vi "ReadEncoder.vi"() -> ()   [LabVIEW 2013]
doc: "This example demonstrates how to use a counter input along with an external clock to continually sample the angular position measured from an encoder.\n\nFor instructions on how to connect your signals to the DAQ device, refer to your device documentation."
uses:
  <vilib>/Utility/error.llb/DialogType.ctl
  <vilib>/DAQmx/read.llb/DAQmx Read (Counter 1D DBL 1Chan NSamp).vi
  <vilib>/DAQmx/create/channels.llb/DAQmx Create Channel (CI-Position-Angular Encoder).vi
  <vilib>/DAQmx/configure/timing.llb/DAQmx Timing (Sample Clock).vi
  <vilib>/DAQmx/create/channels.llb/DAQmx Create Channel (CO-Pulse Generation-Frequency).vi
  <vilib>/DAQmx/configure/timing.llb/DAQmx Timing (Implicit).vi
  <vilib>/DAQmx/miscellaneous.llb/DAQmx Fill In Error Info.vi
  <resource>/objmgr/daqmx.rc
panel:
  out "stop":bool=TRUE
  out "Waveform":waveform(dbl)(graph)={"t0"=timestamp(0 s since 1904-01-01), "dt"=0.001, "Y"=array[16000 elements]}
  out "CO.ActualDutyCycle":dbl=0.5
  out "CO.ActualFreq":dbl=10000.0
  in  "Output Terminal":tag="/Dev1/PFI12"
  in  "CounterOutput":tag="Dev1/ctr1"
  in  "Pulses Per Revolution":u32=200
  in  "EncodeCounterInput":tag="Dev1/ctr0"
  in  "Stop":bool
  in  "Sample Rate":dbl=1000.0
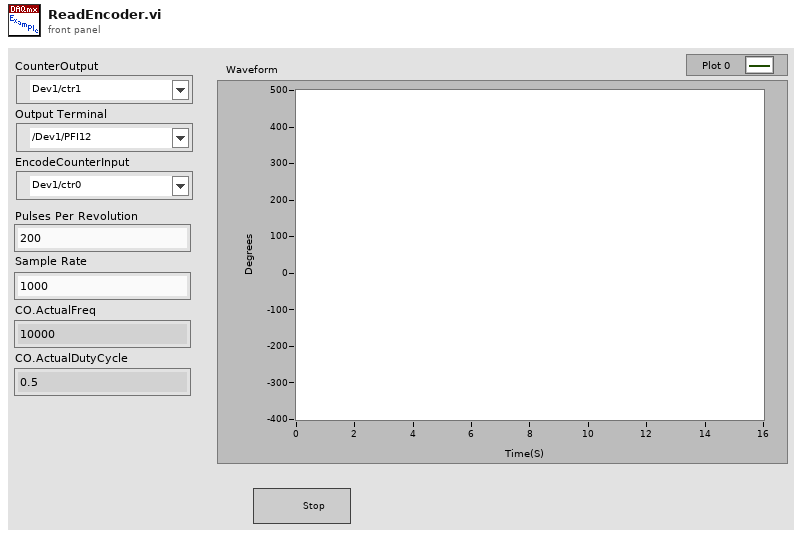
[diagram p1: front panel]
types:
  T1 = typedef "DialogType.ctl" = u16
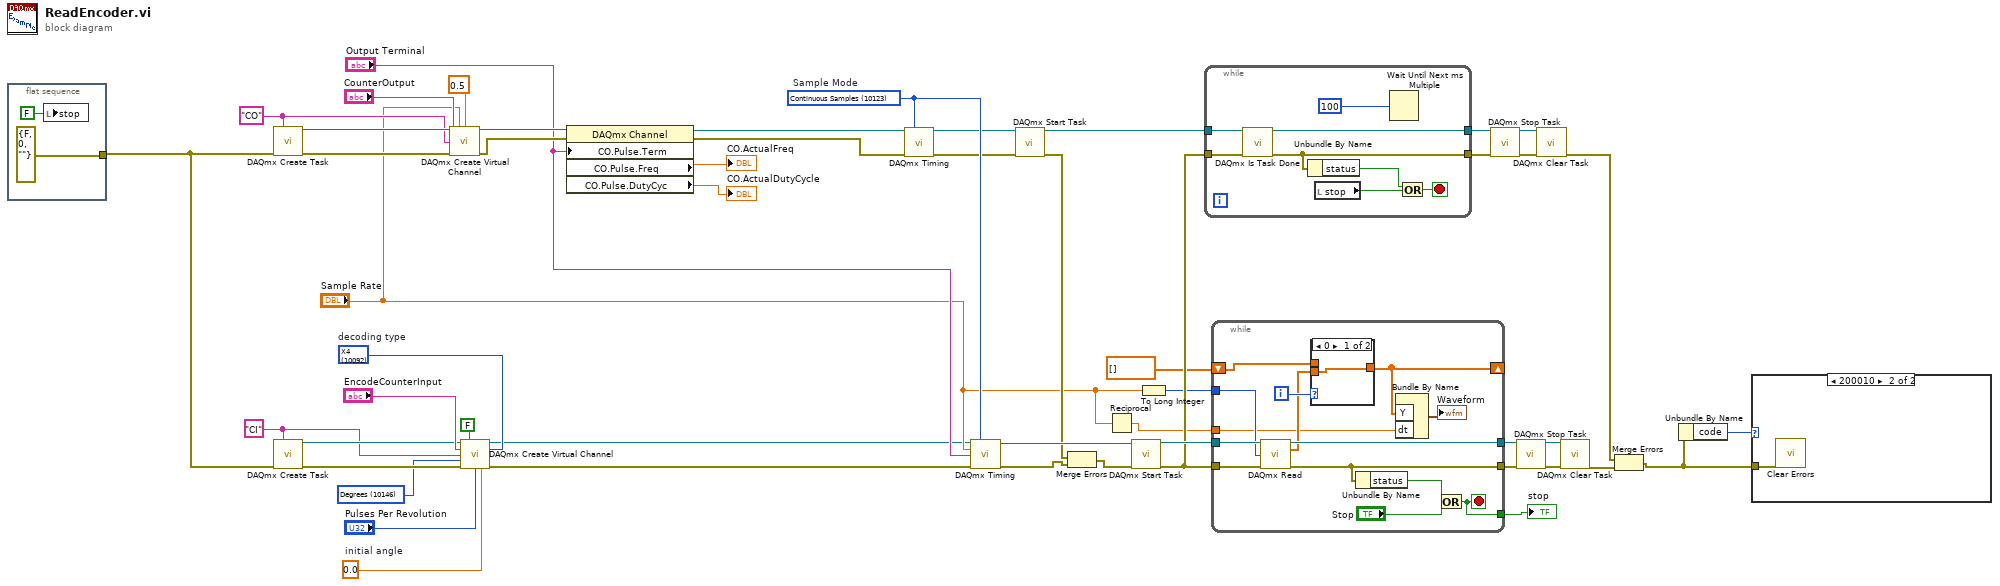
[diagram p0: block diagram]
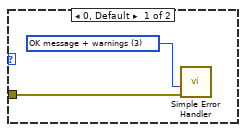
[diagram p2: hidden frame]
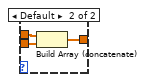
[diagram p3: hidden frame]
diagram:
  w4 = 0.0  # initial angle
  w5 = 10092 items=["X1"=10090, "X2"=10091, "X4"=10092, "Two Pulse Counting"=10313]  # decoding type
  w14 = 10146 items=["Degrees"=10146, "Radians"=10273, "Ticks"=10304, "From Custom Scale"=10065] ("units")
  w15 = "CI" ("new task name")
  w18 = "CO" ("new task name")
  w30 = 10123 items=["Finite Samples"=10178, "Continuous Samples"=10123, "Hardware Timed Single Point"=12522]  # Sample Mode
  n1 = flat-sequence {
    tunnel: [errorcluster {"status"=FALSE, "code"=0, "source"=""} ("error in")] -> w13
    frame #0 {
      n2 = local write "stop"(FALSE ("stop")) -> ()
    }
  }
  n3 = call <vilib>:"DAQmx Create Task.vi"("new task name"=w18, "error in"=w13) -> ("task out"=w20:refnum<k21>, "error out"=w19:errorcluster)  [unwired: 12 in]
  n4 = call <vilib>:"DAQmx Create Task.vi"("new task name"=w15, "error in"=w13) -> ("task out"=w16:refnum<k21>, "error out"=w17:errorcluster)  [unwired: 12 in]
  n5 = call-poly <vilib>:"DAQmx Create Virtual Channel.vi"("task in"=w20, "frequency"="Sample Rate", "duty cycle"=0.5 ("Duty Cycle"), "counter"="CounterOutput", "name to assign"=w18, "error in"=w19) -> ("task out"=w41:refnum<k21>, "error out"=w40:errorcluster)  [unwired: 8 in]
  n6 = call-poly <vilib>:"DAQmx Create Virtual Channel.vi"("task in"=w16, "z index enable"=FALSE ("Z Index Enable"), "counter"="EncodeCounterInput", "decoding type"=w5, "name to assign"=w15, "units"=w14, "error in"=w17, "pulses per revolution"="Pulses Per Revolution", "initial angle"=w4) -> ("task out"=w2:refnum<k21>, "error out"=w1:errorcluster)  [unwired: 5 in]
  n7 = property class="DAQmx Channel"(reference=w41, error in=w40, "CO.Pulse.Term"="Output Terminal") -> (reference out=w38:refnum<k21>, error out=w39:errorcluster, "CO.Pulse.Freq"=→"CO.ActualFreq":dbl, "CO.Pulse.DutyCyc"=→"CO.ActualDutyCycle":dbl)
  n8 = call-poly <vilib>:"DAQmx Timing.vi"("task/channels in"=w38, "sample mode"=w30, "error in"=w39) -> ("task out"=w29:refnum<k21>, "error out"=w28:errorcluster)  [unwired: 11 in]
  n9 = call-poly <vilib>:"DAQmx Timing.vi"("task/channels in"=w2, "sample mode"=w30, "rate"="Sample Rate", "source"="Output Terminal", "error in"=w1) -> ("task out"=w27:refnum<k21>, "error out"=w26:errorcluster)  [unwired: 9 in]
  n10 = call <vilib>:"DAQmx Start Task.vi"("task/channels in"=w29, "error in"=w28) -> ("task out"=w43:refnum<k21>, "error out"=w25:errorcluster)  [unwired: 12 in]
  n11 = Merge Errors(w25, w26) -> (w24:errorcluster)
  n12 = Reciprocal(x="Sample Rate") -> (1/x=w7:dbl)
  n13 = call <vilib>:"DAQmx Start Task.vi"("task/channels in"=w27, "error in"=w24) -> ("task out"=w51:refnum<k21>, "error out"=w23:errorcluster)  [unwired: 12 in]
  n14 = To Long Integer(number="Sample Rate") -> (32bit integer=w22:i32)
  n15 = while {
    tunnel: w43 -> [w61]
    tunnel: w23 -> [w60]
    tunnel: [w57] -> w31
    tunnel: [w58] -> w32
    stop <- w59 stop-if-true
    n16 = call <vilib>:"DAQmx Is Task Done.vi"("task/channels in"=w61, "error in"=w60) -> ("task out"=w58:refnum<k21>, "error out"=w57:errorcluster)  [unwired: 11 in, 1 out]
    n17 = Unbundle By Name(w57) -> ("status"=w56:bool)
    n18 = local read "stop"() -> (w54:bool)
    n19 = Wait Until Next ms Multiple(millisecond multiple=u32 100) -> ()  [unwired: 1 out]
    n20 = Or(x=w56, y=w54) -> (x .or. y?=w59:bool)
  }
  n21 = while {
    tunnel: w51 -> [w75]
    tunnel: w23 -> [w74]
    tunnel: [w72] -> w46
    tunnel: [w73] -> w47
    tunnel: w22 -> [w69]
    tunnel: [w68] -> w21
    shift-right: [w64] -> _
    shift-left: dbl[] [] -> [w65]
    tunnel: w7 -> [w63]
    i -> [w67]
    stop <- w68 stop-if-true
    n22 = call-poly <vilib>:"DAQmx Read.vi"("task/channels in"=w75, "number of samples per channel"=w69, "error in"=w74) -> ("task out"=w73:refnum<k21>, "data"=w66:dbl[], "error out"=w72:errorcluster)  [unwired: 10 in]
    n23 = case shown="0" w67 {
      tunnel: w66 -> [w76 w79]
      tunnel: [w76 w78] -> w64
      tunnel: w65 -> [_ w77]
      frame 0 {
      }
      frame Default {
        n24 = Build Array (concatenate)(w77, w79) -> (w78:dbl[])
      }
    }
    n25 = Unbundle By Name(w72) -> ("status"=w71:bool)
    n26 = Bundle By Name("Y"=w64, "dt"=w63) -> (→"Waveform":waveform(dbl))  [unwired: 1 in]
    n27 = Or(x=w71, y="Stop") -> (x .or. y?=w68:bool)
  }
  "stop" <- w21
  n28 = call <vilib>:"DAQmx Stop Task.vi"("task/channels in"=w32, "error in"=w31) -> ("task out"=w34:refnum<k21>, "error out"=w33:errorcluster)  [unwired: 12 in]
  n29 = call <vilib>:"DAQmx Stop Task.vi"("task/channels in"=w47, "error in"=w46) -> ("task out"=w44:refnum<k21>, "error out"=w45:errorcluster)  [unwired: 12 in]
  n30 = call <vilib>:"DAQmx Clear Task.vi"("task in"=w34, "error in"=w33) -> ("error out"=w10:errorcluster)  [unwired: 13 in]
  n31 = call <vilib>:"DAQmx Clear Task.vi"("task in"=w44, "error in"=w45) -> ("error out"=w11:errorcluster)  [unwired: 13 in]
  n32 = Merge Errors(w10, w11) -> (w9:errorcluster)
  n33 = Unbundle By Name(w9) -> ("code"=w12:i32)
  n34 = case shown="200010" w12 {
    tunnel: w9 -> [w81 w82]
    frame 0, Default {
      w80 = T1 3 items=["no dialog", "OK message", "continue or stop message", "OK message + warnings", "continue/stop + warnings"] ("type of dialog (OK msg:1)")
      n35 = call <vilib>:"Simple Error Handler.vi"("type of dialog (OK msg:1)"=w80, "error in (no error)"=w81) -> ()  [unwired: 3 in, 5 out]
    }
    frame 200010 {
      n36 = call <vilib>:"Clear Errors.vi"("error in (no error)"=w82) -> ()  [unwired: 6 in, 1 out]
    }
  }
